vi "Move Robot to End of Path.vi"(10 "Robot Path":cluster{dbl[], dbl[]}, 11 "Robot Plot":cluster{dbl[], dbl[]}) -> (2 "Robot Position":cluster{"x":dbl, "y":dbl}, 3 "Robot Plot Out":cluster{dbl[], dbl[]})   [LabVIEW 2017]
uses:
  <vilib>/Analysis/coordinate.llb/2D Cartesian Coordinate Rotation (Array).vi
  <vilib>/Analysis/coordinate.llb/2D Cartesian Coordinate Shift (Array).vi
  <vilib>/Analysis/NI_AALPro.lvlib
panel:
  out "Ideal Robot Angle":dbl
  out "XY Graph":cluster{dbl[], dbl[]}[](graph)
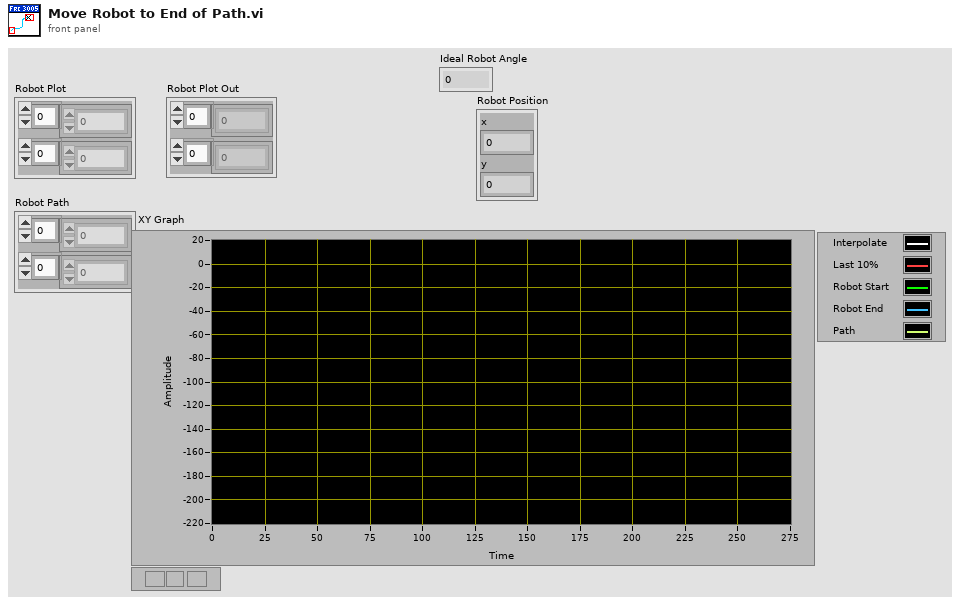
[diagram p1: front panel]
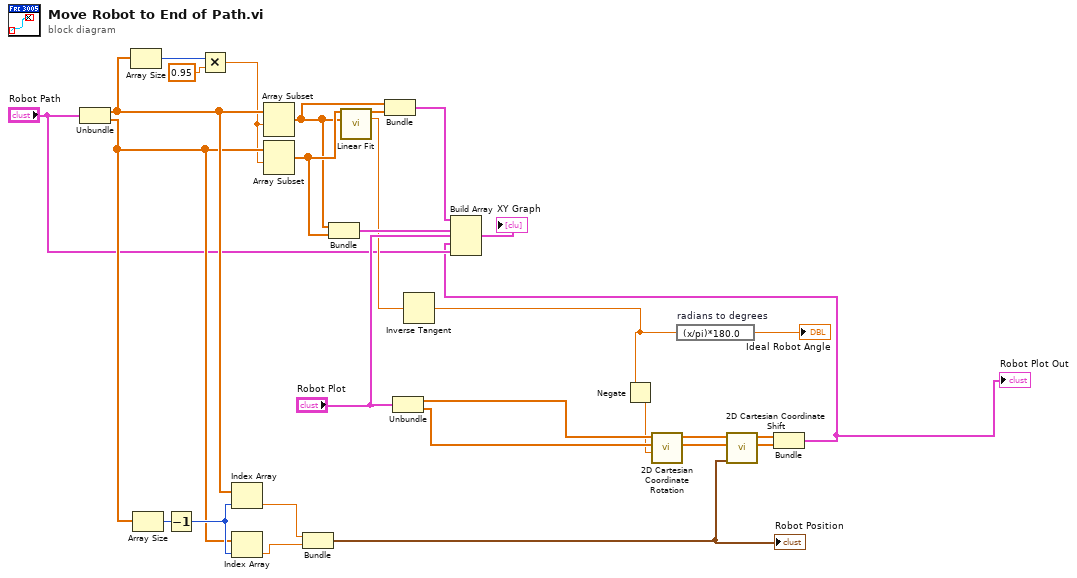
[diagram p0: block diagram]
diagram:
  n1 = Unbundle("Robot Path") -> (w18:dbl[], w17:dbl[])
  n2 = Array Size(array=w18) -> (size(s)=w29:i32)
  n3 = Array Size(array=w17) -> (size(s)=w20:i32)
  n4 = Decrement(x=w20) -> (x-1=w19:i32)
  n5 = Multiply(x=w29, y=0.95) -> (x*y=w7:dbl)
  n6 = Index Array(array=w18, index=w19) -> (element=w14:dbl)
  n7 = Index Array(array=w17, index=w19) -> (element=w15:dbl)
  n8 = Array Subset(array=w18, index=w7) -> (w23:dbl[])  [unwired: 1 in]
  n9 = Array Subset(array=w17, index=w7) -> (w27:dbl[])  [unwired: 1 in]
  n10 = Bundle("x"=w14, "y"=w15) -> (w13:cluster{"x":dbl, "y":dbl})  [unwired: 1 in]
  "Robot Position" <- w13
  n11 = Bundle(w23, w27) -> (w26:cluster{dbl[], dbl[]})  [unwired: 1 in]
  n12 = call <vilib>:"Linear Fit.vi"("Y"=w27, "X"=w23) -> ("Best Linear Fit"=w24:dbl[], "slope"=w12:dbl)  [unwired: 9 in, 3 out]
  n13 = Bundle(w23, "Best Linear Fit"=w24) -> (w22:cluster{dbl[], "Best Linear Fit":dbl[]})  [unwired: 1 in]
  n14 = Unbundle("Robot Plot") -> (w9:dbl[], w21:dbl[])
  n15 = Inverse Tangent(1:w12) -> (0:w11:dbl)
  n16 = Negate(x=w11) -> (-x=w1:dbl)
  n17 = call-poly <vilib>:"2D Cartesian Coordinate Rotation.vi"("theta"=w1, "Y"=w21, "X"=w9) -> ("Y Out"=w5:dbl[], "X Out"=w6:dbl[])  [unwired: 6 in, 1 out]
  n18 = expression code="(x/pi)*180.0" "radians to degrees"(w11) -> (→"Ideal Robot Angle":dbl)
  n19 = call-poly <vilib>:"2D Cartesian Coordinate Shift.vi"("shift"=w13, "Y"=w5, "X"=w6) -> ("Y Out"=w4:dbl[], "X Out"=w3:dbl[])  [unwired: 6 in, 1 out]
  n20 = Bundle("X Out"=w3, "Y Out"=w4) -> (w2:cluster{"X Out":dbl[], "Y Out":dbl[]})  [unwired: 1 in]
  "Robot Plot Out" <- w2
  n21 = Build Array(w22, w26, "Robot Plot", w2, "Robot Path") -> (→"XY Graph":cluster{"X Out":dbl[], "Y Out":dbl[]}[])
